vi "async request safe state.vi"(11 "async execution info in":T1) -> (3 "async execution info out":T1)   [LabVIEW 2013, in "Standard Engine Runtime.lvclass"]
uses:
  Standard Engine Runtime.lvclass
  async execution info.ctl
  asynchronous process data.ctl
  async command notification.ctl
  <vilib>/NI/Tag Bus/table/data table.ctl
  <vilib>/NI/Tag Bus Module Framework/runtime/execution settings.ctl
  async error info.ctl
  <vilib>/NI/Tag Bus Module Framework/runtime/error classification.ctl
  Data Table with Transfer Spec.ctl
  <vilib>/NI/Tag Bus/table/transfer specification.ctl
  <vilib>/NI/Tag Bus/tag/Data Type.ctl
  Configuration/Module Decimation.ctl
  Configuration/Module Error Configuration.ctl
  Configuration/Error Actions By Category.ctl
  Configuration/Error Actions.ctl
  <vilib>/NI/Tag Bus/table/data table.lvlib
  <vilib>/NI/Tag Bus Module Framework/runtime/TBM module execution interface.lvclass
  <vilib>/NI/Tag Bus/tag/tag descriptor.lvclass
  Configuration/Standard Engine Configuration.lvclass
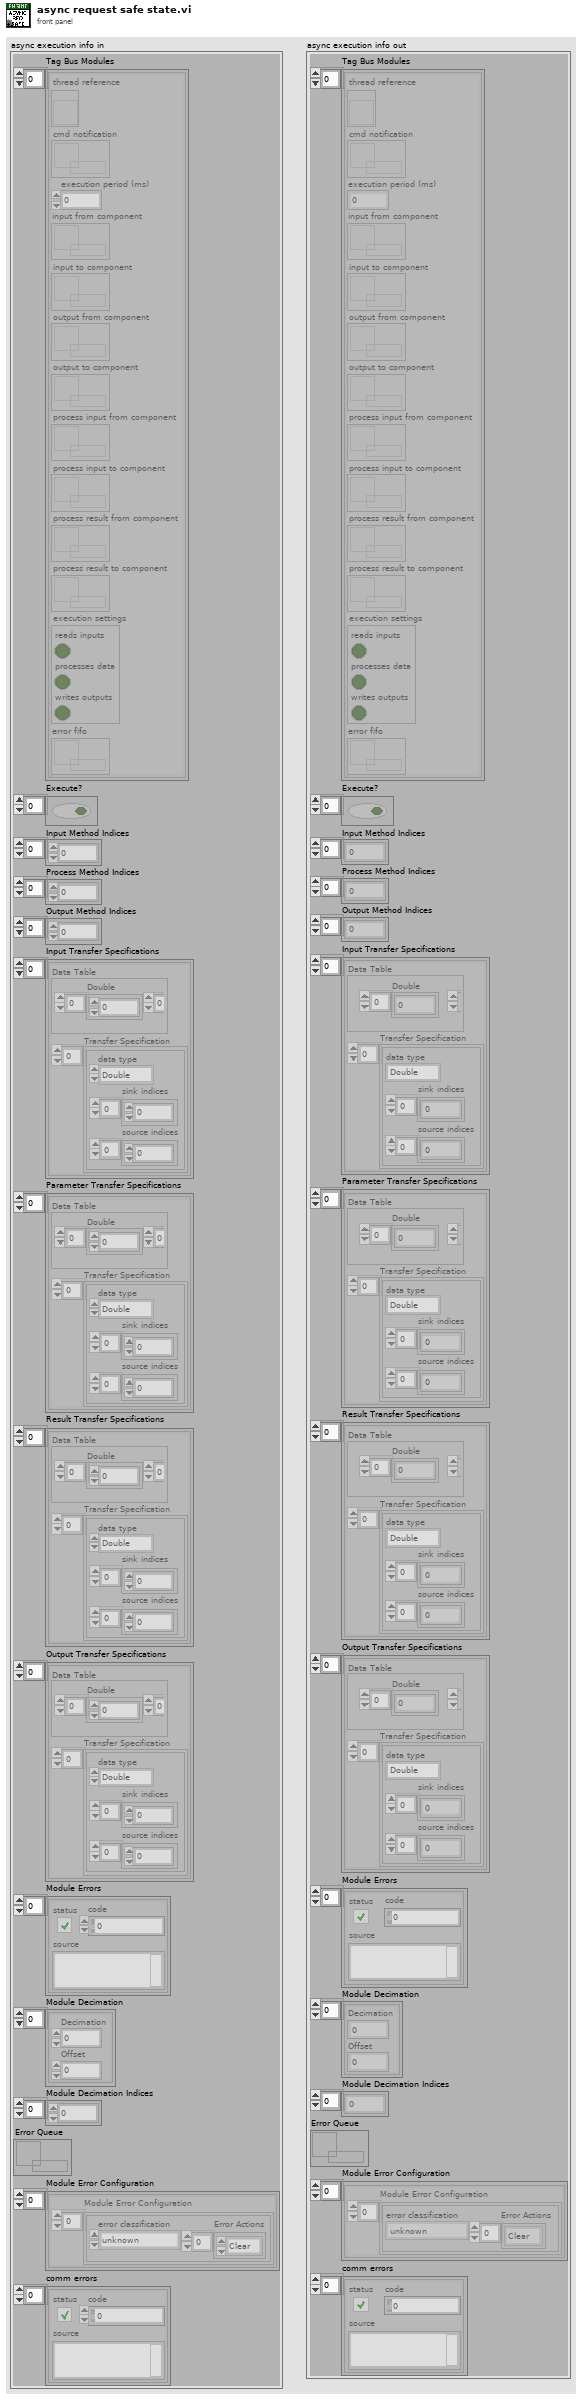
[diagram p1: front panel]
types:
  T1 = typedef "Standard Engine Runtime.lvclass/async execution info.ctl" = cluster{"Tag Bus Modules":T2[], "Execute?":bool[], "Input Method Indices":i32[], "Process Method Indices":i32[], "Output Method Indices":i32[], "Input Transfer Specifications":T4[], "Parameter Transfer Specifications":T4[], "Result Transfer Specifications":T4[], "Output Transfer Specifications":T4[], "Module Errors":errorcluster[], "Module Decimation":T8[], "Module Decimation Indices":i32[], "Error Queue":refnum<queue>, "Module Error Configuration":T9[], "comm errors":errorcluster[]}
  T2 = typedef "Standard Engine Runtime.lvclass/asynchronous process data.ctl" = cluster{"thread reference":refnum<vi>, "cmd notification":refnum<k33>, "execution period (ms)":i32, "input from component":refnum<queue>, "input to component":refnum<queue>, "output from component":refnum<queue>, "output to component":refnum<queue>, "process input from component":refnum<queue>, "process input to component":refnum<queue>, "process result from component":refnum<queue>, "process result to component":refnum<queue>, "execution settings":T3, "error fifo":refnum<k33>}
  T3 = typedef "TBM module execution interface.lvclass/execution settings.ctl" = cluster{"reads inputs":bool, "processes data":bool, "writes outputs":bool}
  T4 = typedef "Standard Engine Runtime.lvclass/Data Table with Transfer Spec.ctl" = cluster{"Data Table":T5, "Transfer Specification":T6[]}
  T5 = typedef "tag bus.lvlib/data table.lvlib/data table.ctl" = cluster{"Double":dbl[], "Single":sgl[], "I64":i64[], "I32":i32[], "I16":i16[], "I8":i8[], "U64":u64[], "U32":u32[], "U16":u16[], "U8":u8[], "Boolean":bool[], "String":string[], "Array of Double":cluster{"DBL Array":dbl[]}[], "Array of Single":cluster{"SGL Array":sgl[]}[], "Array of I64":cluster{"I64 Array":i64[]}[], "Array of I32":cluster{"I32 Array":i32[]}[], "Array of I16":cluster{"I16 Array":i16[]}[], "Array of I8":cluster{"I8 Array":i8[]}[], "Array of U64":cluster{"U64 Array":u64[]}[], "Array of U32":cluster{"U32 Array":u32[]}[], "Array of U16":cluster{"U16 Array":u16[]}[], "Array of U8":cluster{"U8 Array":u8[]}[], "Array of Boolean":cluster{"Boolean Array":bool[]}[], "Array of String":cluster{"String Array":string[]}[]}
  T6 = typedef "tag bus.lvlib/data table.lvlib/transfer specification.ctl" = cluster{"data type":T7, "sink indices":i32[], "source indices":i32[]}
  T7 = typedef "tag bus.lvlib/tag descriptor.lvclass/Data Type.ctl" = enum16{"Double", "Single", "I64", "I32", "I16", "I8", "U64", "U32", "U16", "U8", "Boolean", "String", "Array of Double", "Array of Single", "Array of I64", "Array of I32", "Array of I16", "Array of I8", "Array of U64", "Array of U32", "Array of U16", "Array of U8", "Array of Boolean", "Array of String"}
  T8 = typedef "Standard Engine Configuration.lvclass/Module Decimation.ctl" = cluster{"Decimation":u16, "Offset":u16}
  T9 = typedef "Standard Engine Configuration.lvclass/Module Error Configuration.ctl" = cluster{"Module Error Configuration":T10[]}
  T10 = typedef "Standard Engine Configuration.lvclass/Error Actions By Category.ctl" = cluster{"error classification":T11, "Error Actions":T12[]}
  T11 = typedef "TBM module execution interface.lvclass/error classification.ctl" = enum16{"unknown", "none", "trivial", "recoverable", "critical"}
  T12 = typedef "Standard Engine Configuration.lvclass/Error Actions.ctl" = enum16{"Clear", "Notify", "Stop Component", "Stop Engine", "Safe State", "Attempt Recovery"}
  T13 = typedef "Standard Engine Runtime.lvclass/async command notification.ctl" = enum16{"stop", "safe state", "recover", "clear error"}
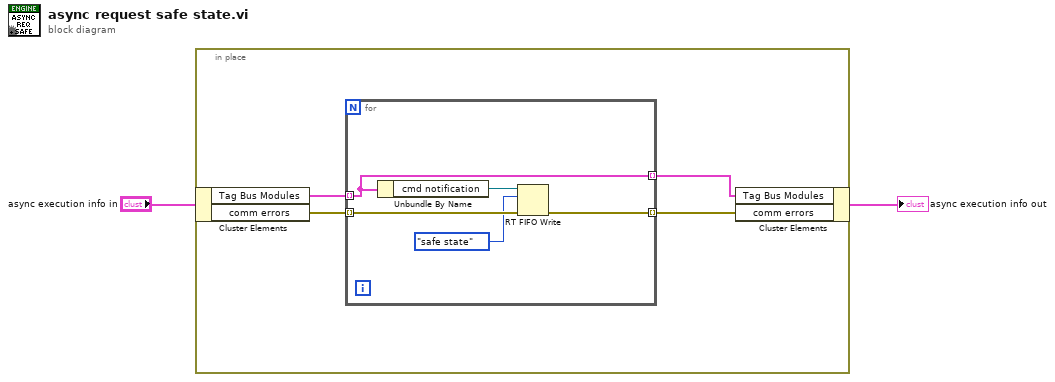
[diagram p0: block diagram]
diagram:
  n1 = in-place {
    n2 = in-place-cluster #1("async execution info in") -> ("Tag Bus Modules"=w5:T2[], "comm errors"=w6:errorcluster[])
    n3 = for {
      tunnel: w5 -> [w7] mode=indexing
      tunnel: w6 -> [w11] mode=indexing
      tunnel: [w10] -> w4 mode=indexing
      tunnel: [w7] -> w3 mode=indexing
      n4 = Unbundle By Name(w7) -> ("cmd notification"=w9:refnum<k33>)
      n5 = RT FIFO Write(0:w9, 1:async_command_notification."safe state" ("element"), 3:w11) -> (11:w10:errorcluster)  [unwired: 2 in, 3 out]
    }
    n6 = in-place-cluster #1("Tag Bus Modules"=w3, "comm errors"=w4) -> (→"async execution info out":T1)
  }
